vi "Read Results from Query TDM.vi"(8 "error in (no error)":errorcluster, 11 "Query Path":path) -> (0 "error out":errorcluster, 3 "Results":string[][](array[string]))   [LabVIEW 2011]
uses:
  <vilib>/Platform/storage/lvStorage.llb/xStorage/Read Data/Read Data.xnode
  <vilib>/Platform/storage/lvStorage.llb/xStorage/Get Properties/Get Properties.xnode
  <vilib>/Platform/storage/lvStorage.llb/_queryPropString.vi
  <vilib>/Platform/storage/lvStorage.llb/_queryGenericObjects.vi
  <vilib>/Platform/storage/lvStorage.llb/xStorage/xStorageSupp/ErrorOut.vi
  <vilib>/Platform/storage/lvStorage.llb/_loadAllString.vi
  <vilib>/Platform/storage/Storage.llb/__loadStringChannel.vi
  <vilib>/Platform/storage/Storage.llb/__loadPropString.vi
panel:
  # "The query passes back an array of [ Filepath, MN, SN, RunID, CHID, Cond1, ... CondN] per row."
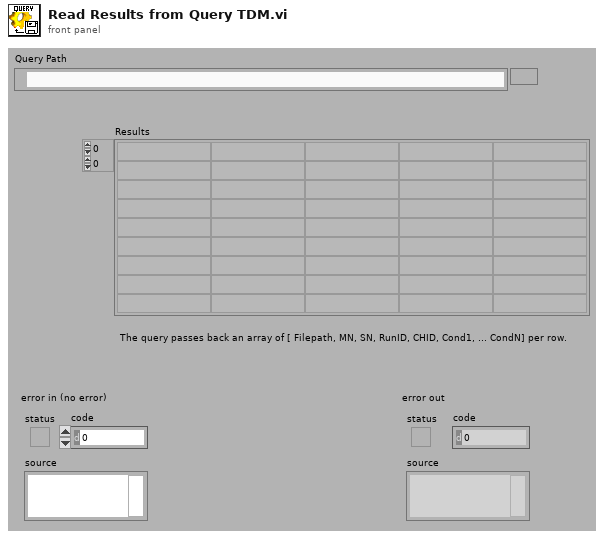
[diagram p1: front panel]
types:
  T1 = enum16{"UPDATE", "READ", "QUERY", "CREATE CHILD", "CREATE", "CONNECT", "DISCONNECT"}
  T2 = enum16{"open", "open or create", "create or replace", "create", "open (read only)"}
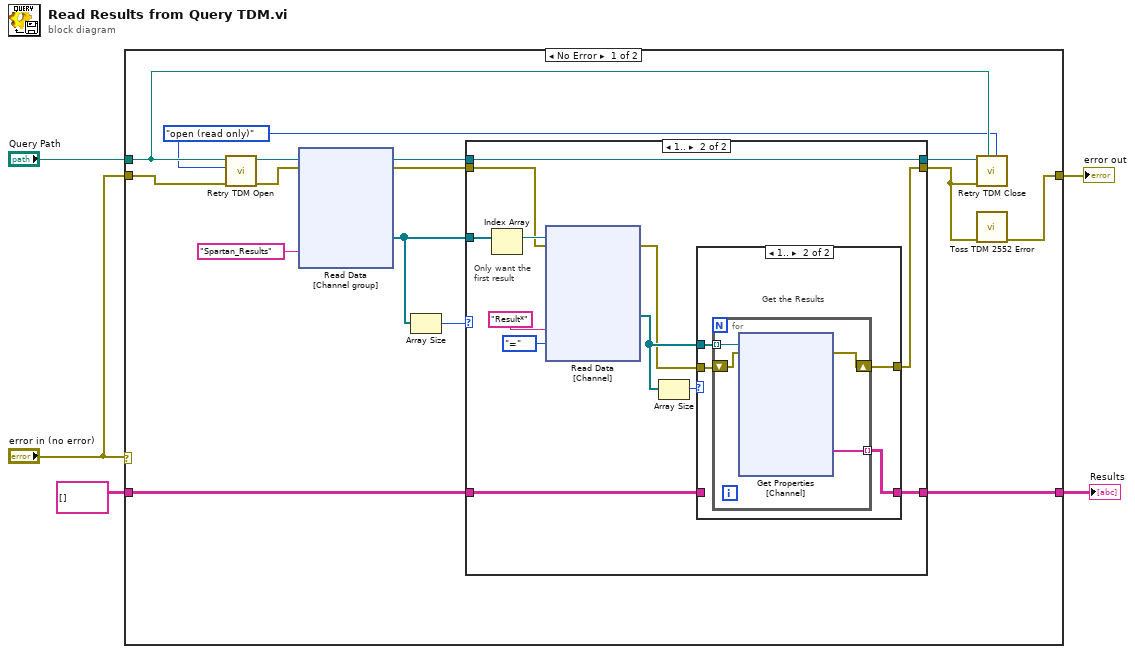
[diagram p0: block diagram]
diagram:
  n1 = case shown="No Error" "error in (no error)" {
    tunnel: "Query Path" -> [w7 _]
    tunnel: "error in (no error)" -> [w10 w94]
    tunnel: [w8 w94] -> w3
    tunnel: string[][] [] ("Signal") -> [w12 w93]
    tunnel: [w11 w93] -> w1
    frame No Error {
      w6 = T2."open (read only)" ("function (open:0)")
      n2 = call "Retry TDM Open.vi"("error in"=w10, "function (open:0)"=w6, "Path"=w7) -> ("error out"=w19:errorcluster, "storage refnum (file)"=w20:refnum<k20>)  [unwired: 7 in]
      n3 = xnode "Read Data\n[Channel group]"("Name"="Spartan_Results", "storage refnum (file)"=w20, "error in"=w19) -> ("storage refnums (channel group)"=w16:refnum<k20>[], "storage refnum (file) out"=w14:refnum<k20>, "error out"=w17:errorcluster)  [unwired: 1 in]
      n4 = Array Size(array=w16) -> (size(s)=w15:i32)
      n5 = case shown="1.." w15 {
        tunnel: [w36 w49] -> w9
        tunnel: w16 -> [_ w48]
        tunnel: w17 -> [w36 w41]
        tunnel: w14 -> [w37 w38]
        tunnel: [w37 w38] -> w13
        tunnel: w12 -> [w35 w40]
        tunnel: [w35 w39] -> w11
        frame 0, Default {
          # "There were no results for this query"
        }
        frame 1.. {
          # "Only want the\nfirst result"
          n6 = Index Array(array=w48) -> (element=w46:refnum<k20>)  [unwired: 1 in]
          n7 = xnode "Read Data\n[Channel]"("Name"="Result*", "Comparison (=)"=enum16{"=", "!=", ">", "<", ">=", "<="}."=", "storage refnum (channel group)"=w46, "error in"=w41) -> ("storage refnums (channel)"=w43:refnum<k20>[], "error out"=w42:errorcluster)  [unwired: 2 out]
          n8 = Array Size(array=w43) -> (size(s)=w47:i32)
          n9 = case shown="1.." w47 {
            tunnel: [w67 w71] -> w49
            tunnel: w43 -> [_ w70]
            tunnel: w42 -> [w67 w69]
            tunnel: w40 -> [w66 _]
            tunnel: [w66 w68] -> w39
            frame 0, Default {
              # "This case shouldn't happen\ntrap it if it does though"
            }
            frame 1.. {
              # "Get the Results"
              n10 = for {
                tunnel: w70 -> [w74] mode=indexing
                tunnel: [w75] -> w68 mode=indexing
                shift-right: [w72] -> w71
                shift-left: w69 -> [w73]
                n11 = xnode "Get Properties\n[Channel]"("storage refnum (channel)"=w74, "error in"=w73) -> ("Signal"=w75:string[], "error out"=w72:errorcluster)  [unwired: 2 in, 3 out]
              }
            }
          }
        }
      }
      n12 = call "Retry TDM Close.vi"("function (open:0)"=w6, "TDM Path"=w7, "error in"=w9, "storage refnum (file)"=w13) -> ()  [unwired: 7 in, 1 out]
      n13 = call "Toss TDM 2552 Error.vi"("error in (no error)"=w9) -> ("error out"=w8:errorcluster)  [unwired: 10 in]
    }
    frame Error {
    }
  }
  "error out" <- w3
  "Results" <- w1
